vi "GetSweepStats.vi"(7 "LabVIEW Web Service Request":refnum<class "Web Request.lvclass">) -> ()   [LabVIEW 2017]
uses:
  <vilib>/wsapi/Web Request.lvclass
  accessors/EmsaWebServiceAccessors.lvlib
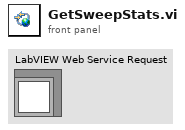
[diagram p1: front panel]
types:
  T1 = typedef "EmsaWebServiceAccessors.lvlib/SweepStats.ctl" = cluster{"Channel":string, "Sweep Time(min)":dbl, "Current Frequency(Hz)":dbl, "Max Sweep Time(min)":dbl, "Completed Sweep":bool}
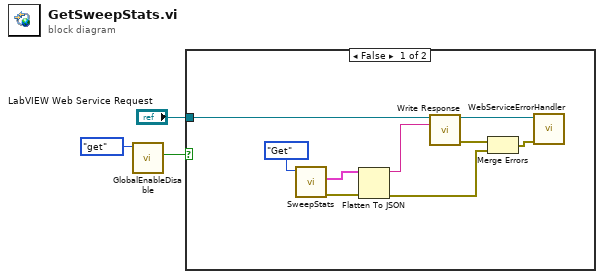
[diagram p0: block diagram]
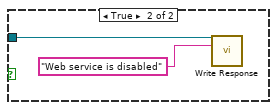
[diagram p2: hidden frame]
diagram:
  n1 = call "GlobalEnableDisable.vi"("action"=enum16{"init", "set", "get"}."get") -> ("DisableDeviceWebService"=w1:bool)  [unwired: 10 in]
  n2 = case shown="False" w1 {
    tunnel: "LabVIEW Web Service Request" -> [w12 w13]
    frame False {
      n3 = call "SweepStats.vi"("Action"=enum16{"Get", "Set"}."Get") -> ("error out"=w4:errorcluster, "sweep stats out"=w5:T1[])  [unwired: 9 in]
      n4 = Flatten To JSON(anything=w5, error in (no error)=w4) -> (JSON string=w8:string, 11:w7:errorcluster)  [unwired: 1 in]
      n5 = call <vilib>:"Write Response.vi"("LabVIEW Web Service Request"=w12, "response string"=w8) -> ("LabVIEW Web Service Request out"=w11:refnum<class "Web Request.lvclass">, "error out"=w10:errorcluster)  [unwired: 12 in]
      n6 = Merge Errors(w10, w7) -> (w9:errorcluster)
      n7 = call "WebServiceErrorHandler.vi"("LabVIEW Web Service Request"=w11, "error in (no error)"=w9) -> ()  [unwired: 12 in, 2 out]
    }
    frame True {
      n8 = call <vilib>:"Write Response.vi"("LabVIEW Web Service Request"=w13, "response string"="Web service is disabled") -> ()  [unwired: 12 in, 2 out]
    }
  }
